vi "Calibration_CreateMatrix.vi"(2 "error in (no error)":errorcluster, 3 "CalibrationCoordinates: x,x',y,y'...":dbl[][](array[numeric])=[[0.0, 0.0, 0.0, 0.0], [1.0, 1.0, 0.0, 0.0], [0.0, 0.0, 1.0, 1.0]]) -> (0 "error out":errorcluster, 1 "Linear conversion Matrix":dbl[][](array[numeric]))   [LabVIEW 2011]
uses:
  <vilib>/Analysis/baseanly.llb/Matrix Type of Inverse Matrix.ctl
  <vilib>/Analysis/7linalg.llb/Solve Linear Equations (single right hand).vi
  <vilib>/Analysis/7linalg.llb/Solve Linear Eqs (General).vi
  <vilib>/Analysis/7linalg.llb/Solve Linear Eqs (Gen, single right hand).vi
  <vilib>/Analysis/NI_AALPro.lvlib
  <vilib>/Analysis/NI_AALBase.lvlib
panel:
  out "size(s)":i32[](array[numeric])
  out "elements":i32
  # "default"
  # "0000\n1100\n0011"
  # "100\n010"
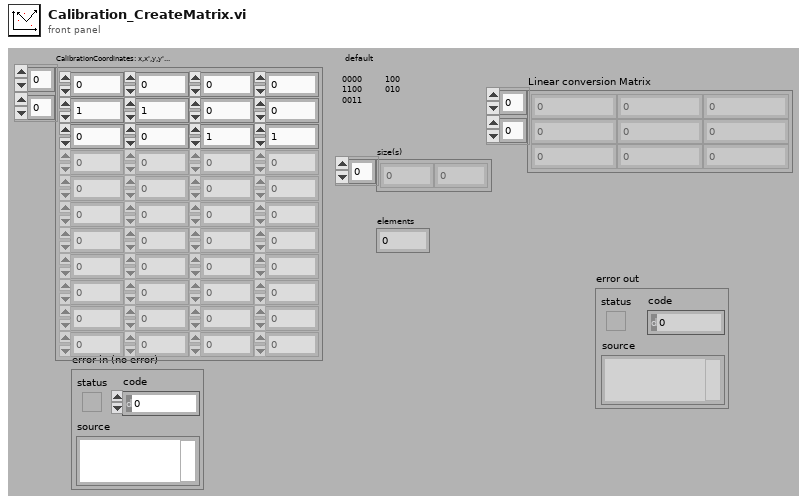
[diagram p1: front panel]
types:
  T1 = typedef "NI_AALBase.lvlib/Matrix Type of Inverse Matrix.ctl" = enum32{"General", "Positive Definite", "Lower Triangular", "Upper Triangular"}
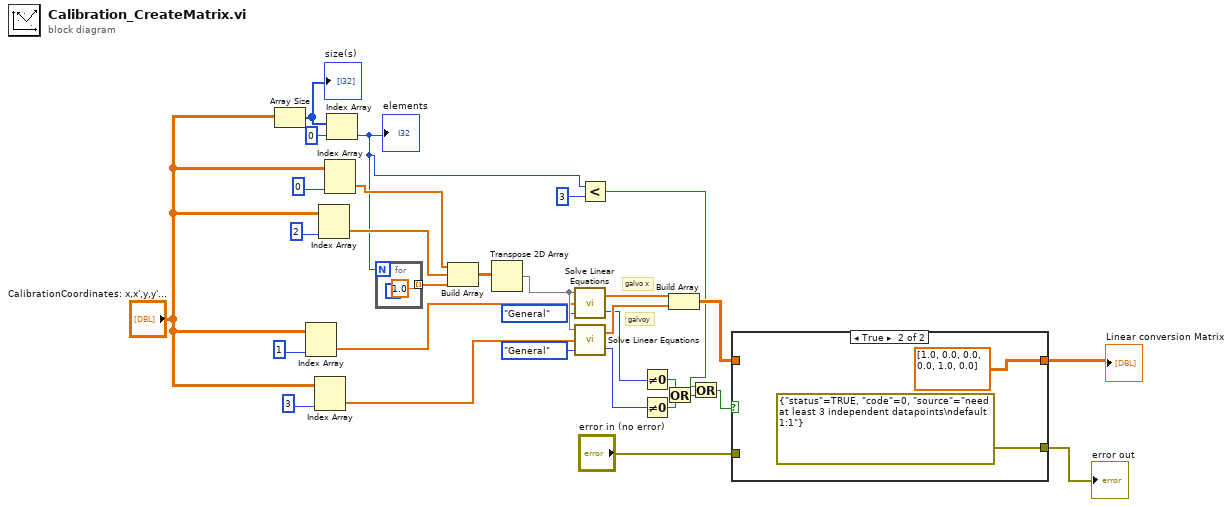
[diagram p0: block diagram]
diagram:
  # "galvoy"
  # "galvo x"
  n1 = Array Size(array="CalibrationCoordinates: x,x',y,y'...") -> (size(s)=w9:i32[])
  "size(s)" <- w9
  n2 = Index Array(array="CalibrationCoordinates: x,x',y,y'...", index (col)=1 ("index (row)")) -> (element=w21:dbl[])  [unwired: 1 in]
  n3 = Index Array(array="CalibrationCoordinates: x,x',y,y'...", index (col)=3 ("index (row)")) -> (element=w20:dbl[])  [unwired: 1 in]
  n4 = Index Array(array="CalibrationCoordinates: x,x',y,y'...", index (col)=2 ("index (row)")) -> (element=w14:dbl[])  [unwired: 1 in]
  n5 = Index Array(array="CalibrationCoordinates: x,x',y,y'...", index (col)=0 ("index (row)")) -> (element=w15:dbl[])  [unwired: 1 in]
  n6 = Index Array(array=w9, index=0) -> (element=w6:i32)
  "elements" <- w6
  n7 = for {
    N: w6 -> [_]
    tunnel: [1.0] -> w29 mode=indexing
  }
  n8 = Build Array(w15, w14, w29) -> (w13:dbl[][])
  n9 = Transpose 2D Array(2D array=w13) -> (transposed array=w28:dbl[][])
  n10 = call-poly <vilib>:"Solve Linear Equations.vi"("matrix type"=Matrix_Type_of_Inverse_Matrix."General", "Known Vector"=w21, "Input Matrix"=w28) -> ("error"=w27:i32, "Solution Vector"=w31:dbl[])
  n11 = call-poly <vilib>:"Solve Linear Equations.vi"("matrix type"=Matrix_Type_of_Inverse_Matrix."General", "Known Vector"=w20, "Input Matrix"=w28) -> ("error"=w26:i32, "Solution Vector"=w30:dbl[])
  n12 = Less?(x=w6, y=3) -> (x < y?=w3:bool)
  n13 = Not Equal To 0?(x=w27) -> (x != 0?=w25:bool)
  n14 = Not Equal To 0?(x=w26) -> (x != 0?=w24:bool)
  n15 = Or(x=w25, y=w24) -> (x .or. y?=w4:bool)
  n16 = Build Array(w31, w30) -> (w12:dbl[][])
  n17 = Or(x=w3, y=w4) -> (x .or. y?=w7:bool)
  n18 = case shown="True" w7 {
    tunnel: "error in (no error)" -> [w34 _]
    tunnel: [w34 errorcluster {"status"=TRUE, "code"=0, "source"="need at least 3 independent datapoints\ndefault 1:1"} ("error in (no error)")] -> w22
    tunnel: w12 -> [w33 _]
    tunnel: [w33 dbl[][] [[1.0, 0.0, 0.0], [0.0, 1.0, 0.0]]] -> w11
    frame False {
    }
    frame True {
    }
  }
  "Linear conversion Matrix" <- w11
  "error out" <- w22
